vi "ReadAttributesTest.vi"() -> ()   [LabVIEW 2009]
uses:
  tango_lv9/tango_vi.llb/avToStringScalarAv.vi
  tango_lv9/tango_vi.llb/avToShortImage.vi
  tango_lv9/tango_vi.llb/avToLongSpectrum.vi
  tango_lv9/tango_vi.llb/avToDoubleScalarAv.vi
  tango_lv9/tango_vi.llb/tango.lvlib
panel:
  out "timestamp":string="sam. 28/01/06 19:14:33,51"
  out "?":string="This is the write value..."
  out "attribute name":string="string_scalar"
  out "quality":string="VALID"
  out "?":i16[][](graph)
  out "?":dbl(graph)
  out "?":i32[](graph)
  out "error stack":string[](array[string])=["no error", "no error", "no error", "read_attributes"]
  out "success":bool=TRUE
  out "error code":i32
  in  "<TangoTest> device name":string="tango/tangotest/1"
  in  "attribute names":string[](array[string])=["double_scalar", "long_spectrum_ro", "short_image_ro", "string_scalar"]
  # "TANGO  Binding for LabVIEW - ReadAttributes example"
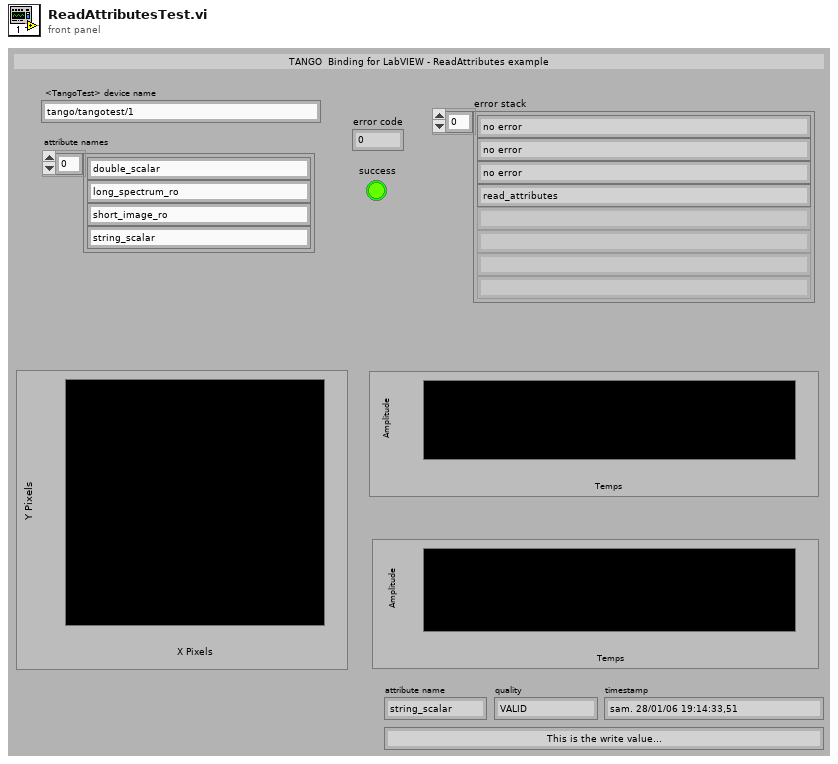
[diagram p1: front panel]
types:
  T1 = cluster{"device name":string, "attribute name":string, "quality value":i16, "quality string":string, "timestamp":dbl, "dim. x":i32, "dim. y":i32, "value":u8[], "error code":i32, "error stack":string[], "data type":enum16{"SCA_STATE", "SCA_STRING", "SPE_STRING", "IMG_STRING", "SCA_BOOLEAN", "SPE_BOOLEAN", "IMG_BOOLEAN", "SCA_UCHAR", "SPE_UCHAR", "IMG_UCHAR", "SCA_SHORT", "SPE_SHORT", "IMG_SHORT", "SCA_USHORT", "SPE_USHORT", "IMG_USHORT", "SCA_LONG", "SPE_LONG", "IMG_LONG", "SCA_ULONG", "SPE_ULONG", "IMG_ULONG", "SCA_FLOAT", "SPE_FLOAT", "IMG_FLOAT", "SCA_DOUBLE", "SPE_DOUBLE", "IMG_DOUBLE", "UNKNOWN_TYPE"}}[]
  T2 = cluster{"device name":string, "attribute name":string, "quality value":i16, "quality string":string, "timestamp":dbl, "dim. x":i32, "dim. y":i32, "value":u8[], "error code":i32, "error stack":string[], "data type":enum16{"SCA_STATE", "SCA_STRING", "SPE_STRING", "IMG_STRING", "SCA_BOOLEAN", "SPE_BOOLEAN", "IMG_BOOLEAN", "SCA_UCHAR", "SPE_UCHAR", "IMG_UCHAR", "SCA_SHORT", "SPE_SHORT", "IMG_SHORT", "SCA_USHORT", "SPE_USHORT", "IMG_USHORT", "SCA_LONG", "SPE_LONG", "IMG_LONG", "SCA_ULONG", "SPE_ULONG", "IMG_ULONG", "SCA_FLOAT", "SPE_FLOAT", "IMG_FLOAT", "SCA_DOUBLE", "SPE_DOUBLE", "IMG_DOUBLE", "UNKNOWN_TYPE"}}
  T3 = cluster{"device name":string, "attribute name":string, "quality value":i16, "quality string":string, "timestamp":dbl, "dim. x":i32, "dim. y":i32, "value":string, "setpoint":string, "error code":i32, "error stack":string[]}
  T4 = cluster{"device name":string, "attribute name":string, "quality value":i16, "quality string":string, "timestamp":dbl, "dim. x":i32, "dim. y":i32, "value":dbl, "error code":i32, "error stack":string[]}
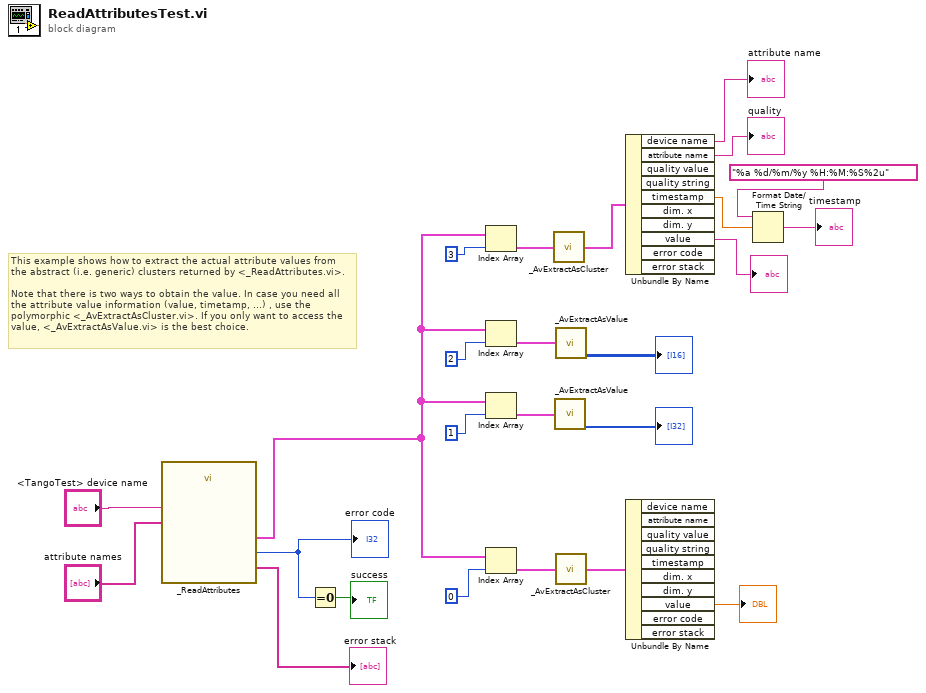
[diagram p0: block diagram]
diagram:
  # "This example shows how to extract the actual attribute values from the abstract (i.e. generic) clusters returned by <_ReadAttributes.vi>. \n\nNote that there is two ways to obtain the value. In case you need all the attribute value information (value, timetamp, ...) , use the polymorphic <_AvExtractAsCluster.vi>. If you only want to access the value, <_AvExtractAsValue.vi> is the best choice."
  n1 = call "_ReadAttributes.vi"("device name"="<TangoTest> device name", "attribute names"="attribute names") -> ("values"=w25:T1, "error code"=w22:i32, "error stack"=→"error stack":string[])
  "error code" <- w22
  n2 = Equal To 0?(x=w22) -> (x = 0?=→"success":bool)
  n3 = Index Array(array=w25, index=3 ("indice")) -> (element=w2:T2)
  n4 = Index Array(array=w25, index=2 ("indice")) -> (element=w1:T2)
  n5 = Index Array(array=w25, index=1 ("indice")) -> (element=w8:T2)
  n6 = Index Array(array=w25, index=0 ("indice")) -> (element=w6:T2)
  n7 = call-poly "_AvExtractAsCluster.vi"("attribute value"=w2) -> ("av"=w13:T3)
  n8 = call-poly "_AvExtractAsValue.vi"("attribute value"=w8) -> ("value"=→"?":i32[])  [unwired: 4 out]
  n9 = call-poly "_AvExtractAsValue.vi"("attribute value"=w1) -> ("value"=→"?":i16[][])  [unwired: 4 out]
  n10 = call-poly "_AvExtractAsCluster.vi"("attribute value"=w6) -> ("av"=w7:T4)
  n11 = Unbundle By Name(w13) -> ("device name"=→"attribute name":string, "attribute name"=→"quality":string, "timestamp"=w10:dbl, "value"=→"?":string)  [unwired: 6 out]
  n12 = Unbundle By Name(w7) -> ("value"=→"?":dbl)  [unwired: 9 out]
  n13 = Format Date/Time String(time format string (%c)="%a %d/%m/%y %H:%M:%S%2u" ("chaîne de format de l'heure (%c)"), seconds (now)=w10) -> (date/time string=→"timestamp":string)  [unwired: 1 in]
